vi "Create PWM Waveform.vi"(6 "Channel Ident":string, 8 "error in":errorcluster, 9 "Duty Cycle":dbl=10.0 format="%0.2p %", 10 "Frequency":dbl=10.0 format="%0.2p Hz", 11 "DO DAQmx Fixed Freq PWM CFG in":refnum<class "DO DAQmx Fixed Freq PWM CFG.lvclass">) -> (0 "error out":errorcluster, 1 "PWM Waveform":digitalwaveform(waveform), 2 "Channel Ident out":string, 3 "DO DAQmx Fixed Freq PWM CFG out":refnum<class "DO DAQmx Fixed Freq PWM CFG.lvclass">)   [LabVIEW 2023, in "DO DAQmx Fixed Freq PWM CFG.lvclass"]
uses:
  DO DAQmx Fixed Freq PWM CFG.lvclass
  Configuration/Configuration JSON/Configuration JSON Base/CFG JSON.lvclass/CFG JSON.ctl
  DO DAQmx Fixed Freq PWM CFG.lvclass/DO DAQmx Fixed Freq PWM CFG.ctl
  501ba0a0-c2c9-46ab-a0a9-86892fbf8d4b.vi
  <vilib>/JDP Science/JSONtext/Find Item.vi
  <vilib>/JDP Science/JSONtext/Next JSON Value.vi
  <vilib>/JDP Science/JSONtext/String Subset.vi
  <vilib>/JDP Science/JSONtext/Parsing/Advance past next JSON Value (inlined COPY).vi
  <vilib>/JDP Science/JSONtext/Parsing/Advance past whitespace.vi
  <vilib>/JDP Science/JSONtext/Parsing/Advance past String.vi
  <vilib>/JDP Science/JSONtext/Parsing/Advance past Number.vi
  <vilib>/JDP Science/JSONtext/Parsing/Advance past Line Ending.vi
  <vilib>/JDP Science/JSONtext/Parsing/Parse Full Path or Item Name.vi
  <vilib>/JDP Science/JSONtext/Parsing/Advance past Array.vi
  <vilib>/JDP Science/JSONtext/Parsing/Advance past Object.vi
  <vilib>/JDP Science/JSONtext/support/Error Cluster From Code.vi
  <vilib>/JDP Science/JSONtext/Offset/Find Item Locations by Path.vi
  <vilib>/JDP Science/JSONtext/JSON text to Variant.vi
  <vilib>/Utility/error.llb/Error Cluster From Error Code.vi
  <vilib>/JDP Science/JSONtext/LVClass Serializer/JSONtext LVClass Serializer.lvclass
  <vilib>/ErrorRing/Error Ring.xnode
  Configuration/Configuration JSON/Configuration JSON Base/CFG JSON.lvclass
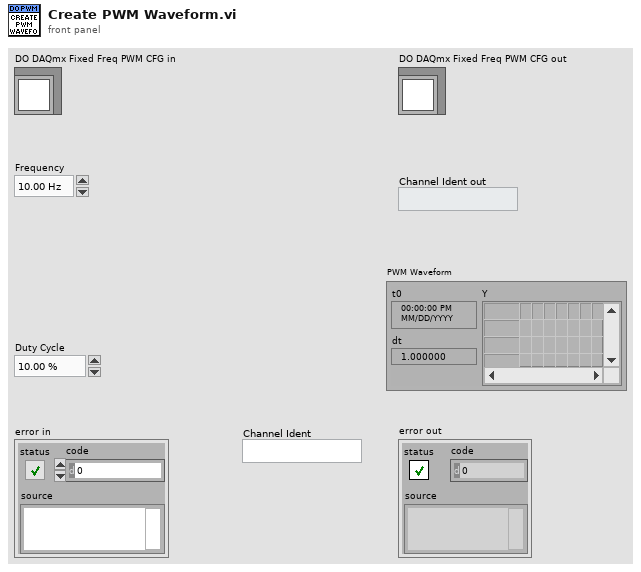
[diagram p1: front panel]
types:
  T1 = cluster{"Samples per Channel":i32, "Sample Rate":dbl}
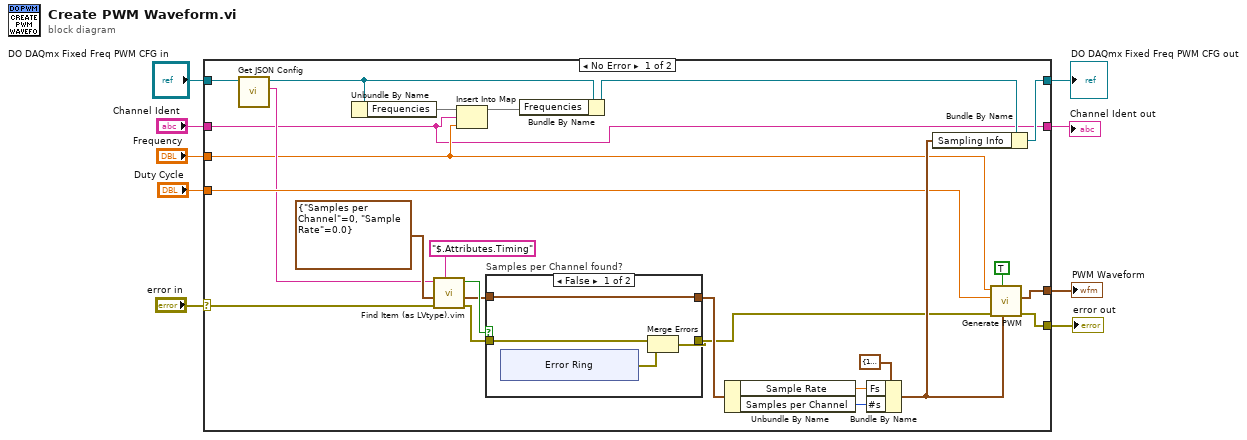
[diagram p0: block diagram]
diagram:
  n1 = case shown="No Error" "error in" {
    selector: "error in" -> [w11 w47]
    tunnel: [w28 _] -> w9
    tunnel: [w27 w47] -> w8
    tunnel: [w23 w48] -> w7
    tunnel: "Frequency" -> [w16 _]
    tunnel: "Duty Cycle" -> [w21 _]
    tunnel: "DO DAQmx Fixed Freq PWM CFG in" -> [w20 w48]
    tunnel: "Channel Ident" -> [w12 w46]
    tunnel: [w12 w46] -> w1
    frame No Error {
      n2 = call "Get JSON Config.vi"("CFG Base in"=w20) -> ("<JSON>Config>"=w19:string, "CFG Base out"=w14:refnum<class "DO DAQmx Fixed Freq PWM CFG.lvclass">)  [unwired: 9 in]
      n3 = Unbundle By Name(w14) -> ("Frequencies"=w17:map{string, dbl})
      n4 = call "Find Item (as LVtype).vim"("$Path or Item Name"="$.Attributes.Timing", "error in (no error)"=w11, "Data Type and Default Value"=T1 {"Samples per Channel"=0, "Sample Rate"=0.0}, "JSON"=w19) -> ("error out"=w33:errorcluster, "Data"=w32:T1, "Found"=w34:bool)  [unwired: 4 in, 1 out]
      n5 = Insert Into Map(map in=w17, key=w12, value=w16) -> (map out=w15:map{string, dbl})  [unwired: 2 out]
      n6 = case "Samples per Channel found?" shown="False" w34 {
        tunnel: w33 -> [w37 w45]
        tunnel: [w36 w45] -> w18
        tunnel: w32 -> [w35 w44]
        tunnel: [w35 w44] -> w29
        frame False {
          n7 = xnode "Error Ring"() -> ("error out"=w38:errorcluster)
          n8 = Merge Errors(w37, w38) -> (w36:errorcluster)
        }
        frame True {
        }
      }
      n9 = Bundle By Name(cluster=w14, "Frequencies"=w15) -> (w13:refnum<class "DO DAQmx Fixed Freq PWM CFG.lvclass">)
      n10 = Unbundle By Name(w29) -> ("Sample Rate"=w25:dbl, "Samples per Channel"=w24:i32)
      n11 = Bundle By Name(cluster=cluster{"Fs":dbl, "#s":dbl} {"Fs"=1000.0, "#s"=1000.0} ("sampling info"), "Fs"=w25, "#s"=w24) -> (w22:cluster{"Fs":dbl, "#s":dbl})
      n12 = Bundle By Name(cluster=w13, "Sampling Info"=w22) -> (w23:refnum<class "DO DAQmx Fixed Freq PWM CFG.lvclass">)
      n13 = call "Generate PWM.vi"("sampling info"=w22, "reset?"=TRUE, "error in"=w18, "duty cycle"=w21, "frequency"=w16) -> ("error out"=w27:errorcluster, "digital waveform"=w28:digitalwaveform)  [unwired: 5 in]
    }
    frame Error {
    }
  }
  "PWM Waveform" <- w9
  "error out" <- w8
  "DO DAQmx Fixed Freq PWM CFG out" <- w7
  "Channel Ident out" <- w1
